vi "Set and Measure ISTR.vi"(4 "Header":string="HighVsec", 5 "String":string, 6 "Name":string, 7 "Position in":u32, 8 "error in (no error)":errorcluster, 9 "Measurement Wait Time":u32, 10 "Cree Comms in":refnum<class "Cree Communications.lvclass">, 11 "Calibration in":refnum<class "Calibration.lvclass">) -> (0 "error out":errorcluster, 2 "DSpic Measurement":dbl, 3 "Actual Measurement":dbl)   [LabVIEW 2015, in "Calibration.lvclass"]
uses:
  Calibration.lvclass
  Classes/Cree Communications/Class/Cree Communications.lvclass
  Test Class/Test Class.lvclass
  Classes/Cree Communications/Cree Comms Messages/CC Message/CC Message.lvclass
  Classes/Cree Communications/Cree Comms Messages/Set Current Reference/Set String Current Ref.lvclass
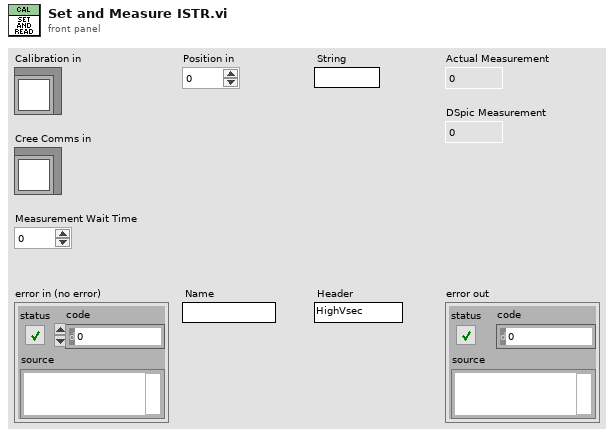
[diagram p1: front panel]
types:
  T1 = cluster{"Current Reference":dbl, "String":enum16{"Red", "BSY1", "BSY2"}}
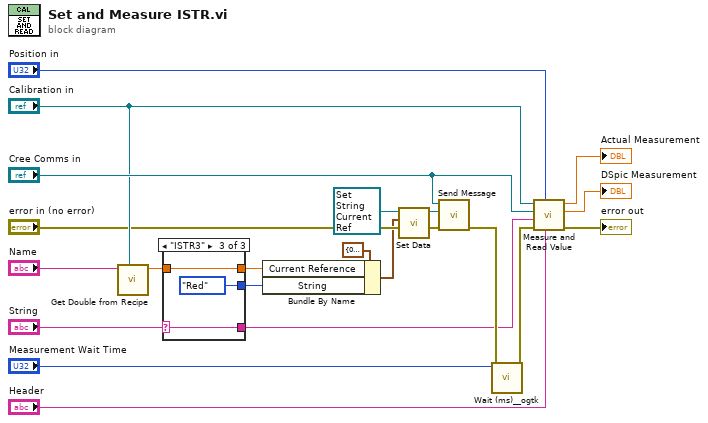
[diagram p0: block diagram]
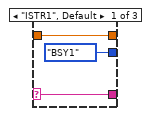
[diagram p2: hidden frame]
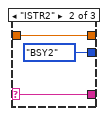
[diagram p3: hidden frame]
diagram:
  n1 = call "Get Double from Recipe.vi"("Test Class in"="Calibration in", "Name"="Name") -> ("Value"=w6:dbl)  [unwired: 7 in, 2 out]
  n2 = case shown="\"ISTR3\"" "String" {
    selector: "String" -> [w23 w26 w29]
    tunnel: w6 -> [w24 w27 w30]
    tunnel: [w24 w27 w30] -> w3
    tunnel: [w23 w26 w29] -> w5
    tunnel: [enum16{"Red", "BSY1", "BSY2"}."BSY1" ("String") enum16{"Red", "BSY1", "BSY2"}."BSY2" ("String") enum16{"Red", "BSY1", "BSY2"}."Red" ("String")] -> w1
    frame "ISTR1", Default {
    }
    frame "ISTR2" {
    }
    frame "ISTR3" {
    }
  }
  n3 = Bundle By Name(cluster=T1 {"Current Reference"=0.0, "String"=enum."Red"} ("Message Type"), "Current Reference"=w3, "String"=w1) -> (w2:T1)
  n4 = call "Set Data.vi"("Data"=w2, "CC Message in"=refnum<class "Set String Current Ref.lvclass"> refnum ("Cree Comms Messages.lvlib:Set String Current Ref.lvclass")) -> ("CC Message out"=w13:refnum<class "Set String Current Ref.lvclass">)  [unwired: 8 in, 1 out]
  n5 = call "Send Message.vi"("error in (no error)"="error in (no error)", "Cree Comms Message"=w13, "Acrobat Template in"="Cree Comms in") -> ("error out"=w15:errorcluster)  [unwired: 7 in, 1 out]
  n6 = call <userlib>:"Wait (ms)__ogtk.vi"("error in (no error)"=w15, "milliseconds to wait"="Measurement Wait Time") -> ("error out"=w16:errorcluster)  [unwired: 8 in, 1 out]
  n7 = call "Measure and Read Value.vi"("Header"="Header", "Position"="Position in", "error in (no error)"=w16, "Calibration Type"=w5, "Cree Communications"="Cree Comms in", "Calibration in"="Calibration in") -> ("error out"=→"error out":errorcluster, "DSpic Measurement"=→"DSpic Measurement":dbl, "Actual Measurement"=→"Actual Measurement":dbl)  [unwired: 3 in]
